vi "ProyectoEstacionamientoFINAL.vi"() -> ()   [LabVIEW 2020]
uses:
  <vilib>/Instr/_visa.llb/VISA Configure Serial Port (Instr).vi
panel:
  out "Lugar  6":string
  out "Lugar 5":string
  out "Lugar 4":string
  out "Lugar 3":string
  out "Lugar 2":string
  out "Lugar 1":string
  out "ESTACIONAMIENTO LLENO":bool
  out "Lugares ocupados":i32
  in  "SALIDA":bool
  in  "ENTRADA":bool
  in  "length (rest) 6":i32
  in  "offset (0) 6":i32
  out "Ocupación espacio 6":string
  out "cadena 6":dbl
  in  "length (rest) 5":i32
  in  "offset (0) 5":i32
  out "Ocupación espacio 5":string
  out "cadena 5":dbl
  in  "length (rest) 4":i32
  in  "offset (0) 4":i32
  out "Ocupación espacio 4":string
  out "cadena 4":dbl
  out "Ocupación espacio 3":string
  in  "length (rest) 3":i32
  in  "offset (0) 3":i32
  out "cadena 3":dbl
  in  "length (rest) 2":i32
  in  "offset (0) 2":i32
  out "Ocupación espacio 2":string
  out "cadena 2":dbl
  out "Ocupación espacio 1":string
  in  "length (rest)":i32
  in  "offset (0)":i32
  out "cadena 1":dbl
  in  "stop":bool
  in  "VISA resource name":refnum<visa-resource-name>
  # "Bienvenidos al estacionamiento de la UPIIZ"
  # "Toca el botón para continuar"
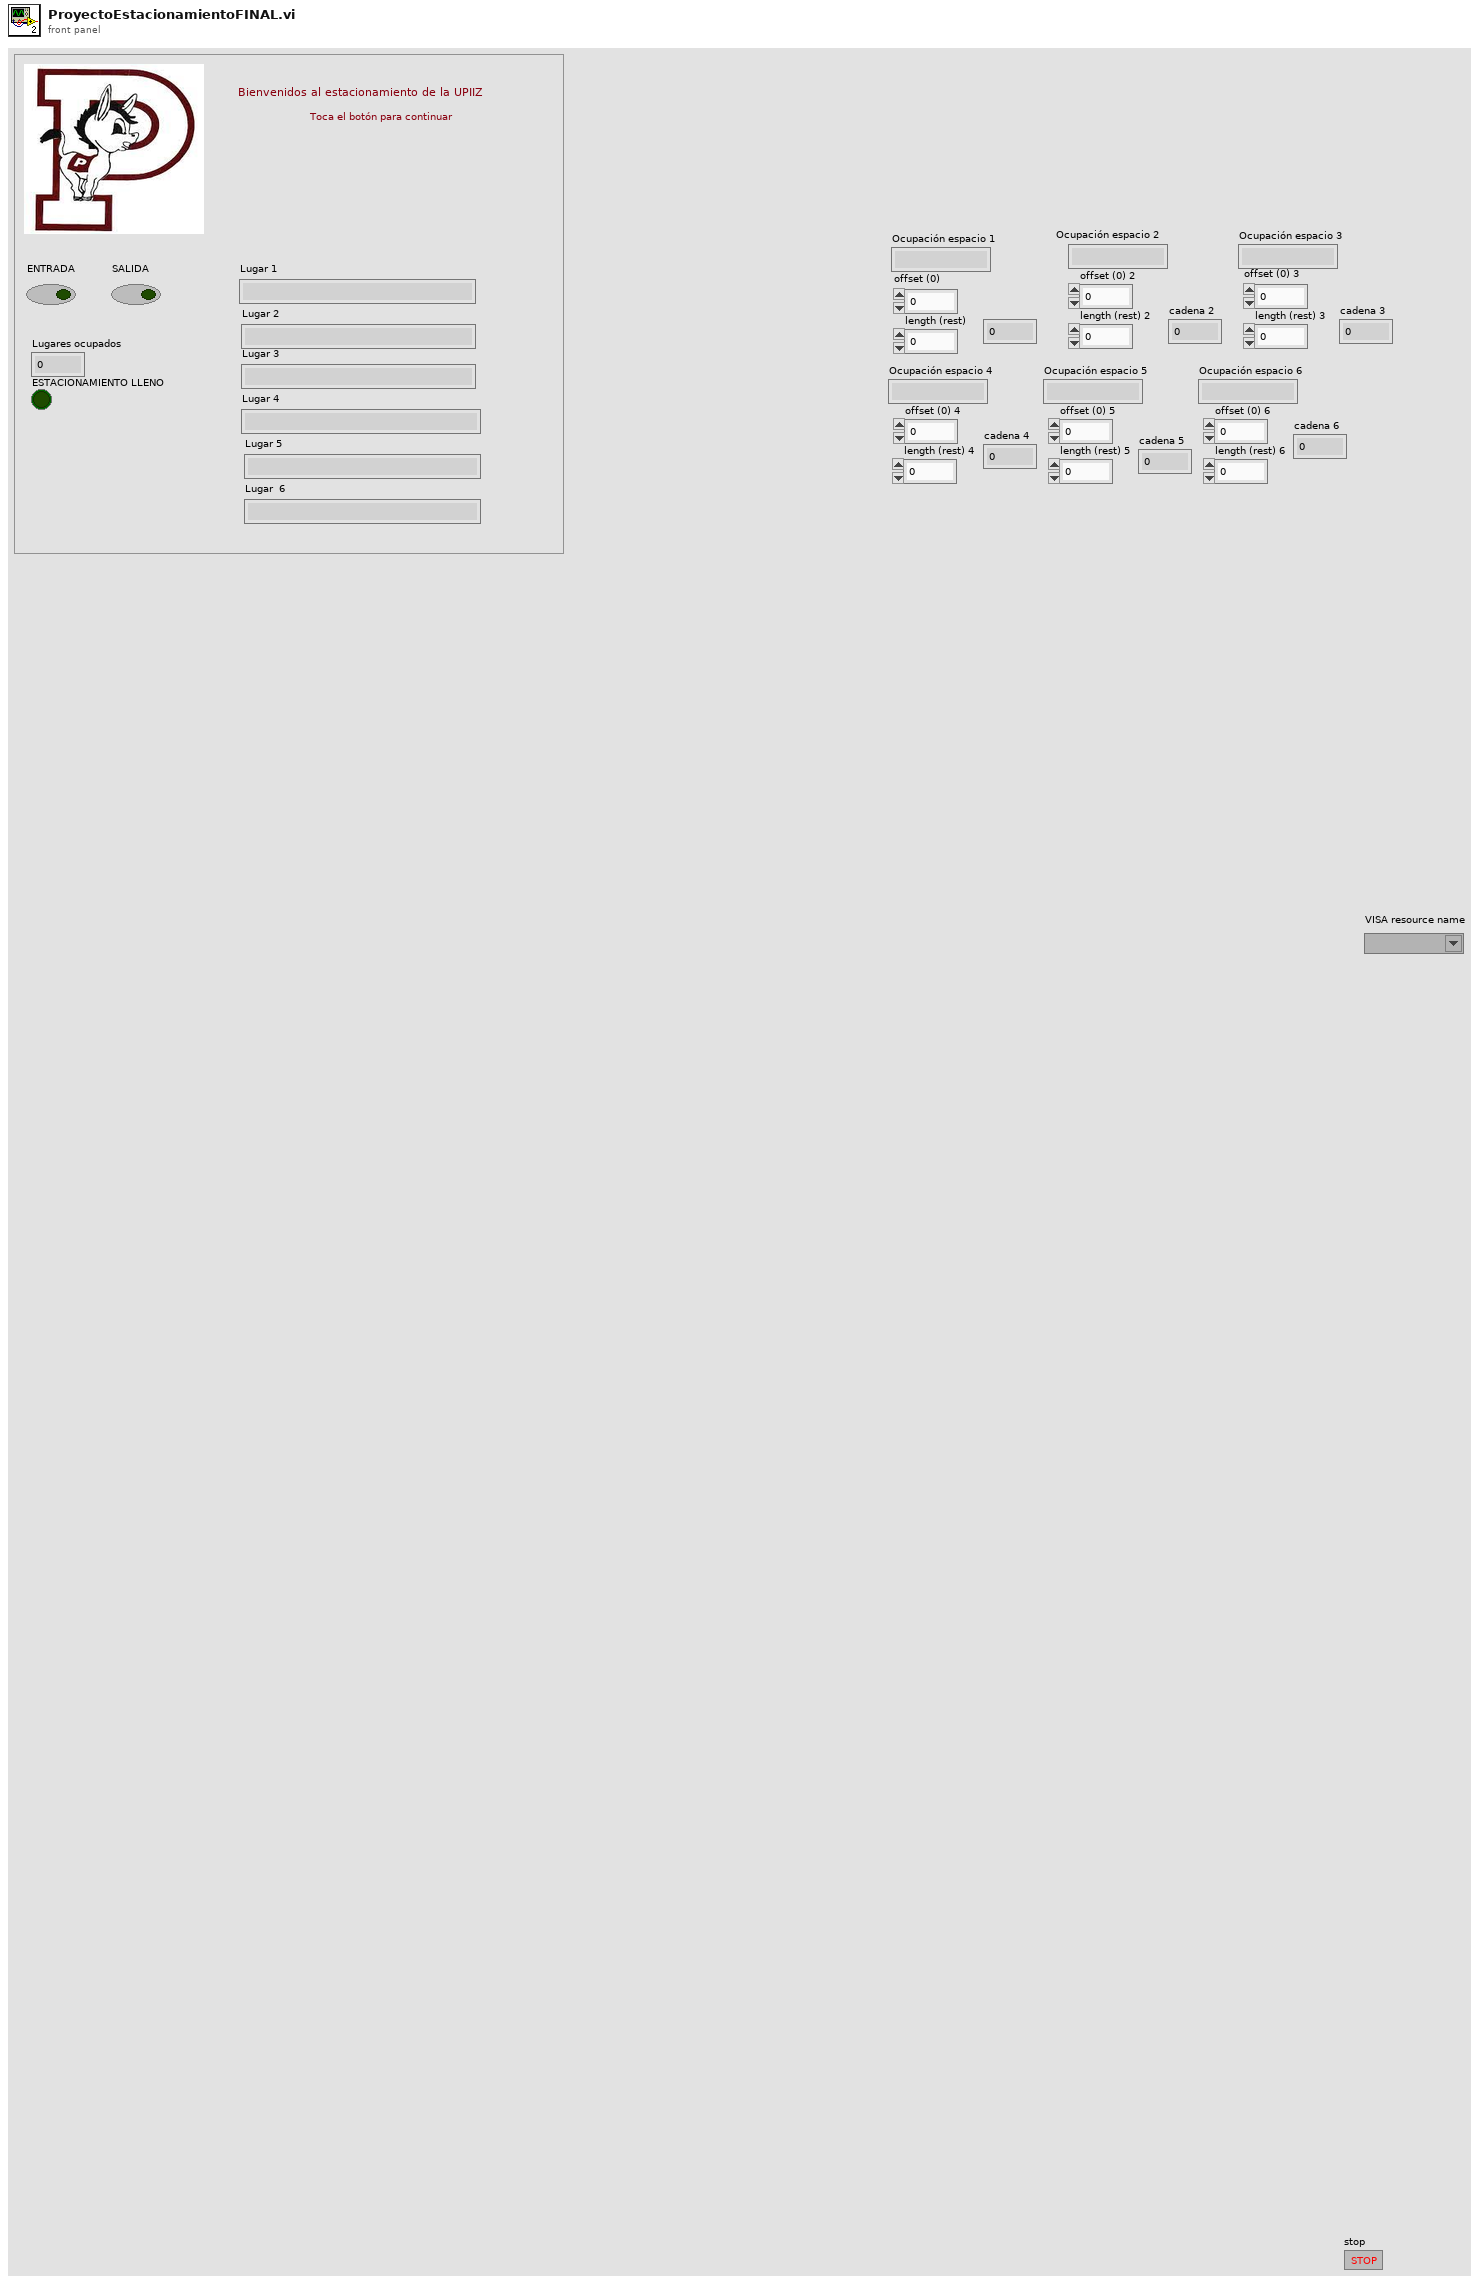
[diagram p1: front panel]
types:
  T1 = enum8{"Enabled", "Disabled", "Disabled and Grayed Out"}
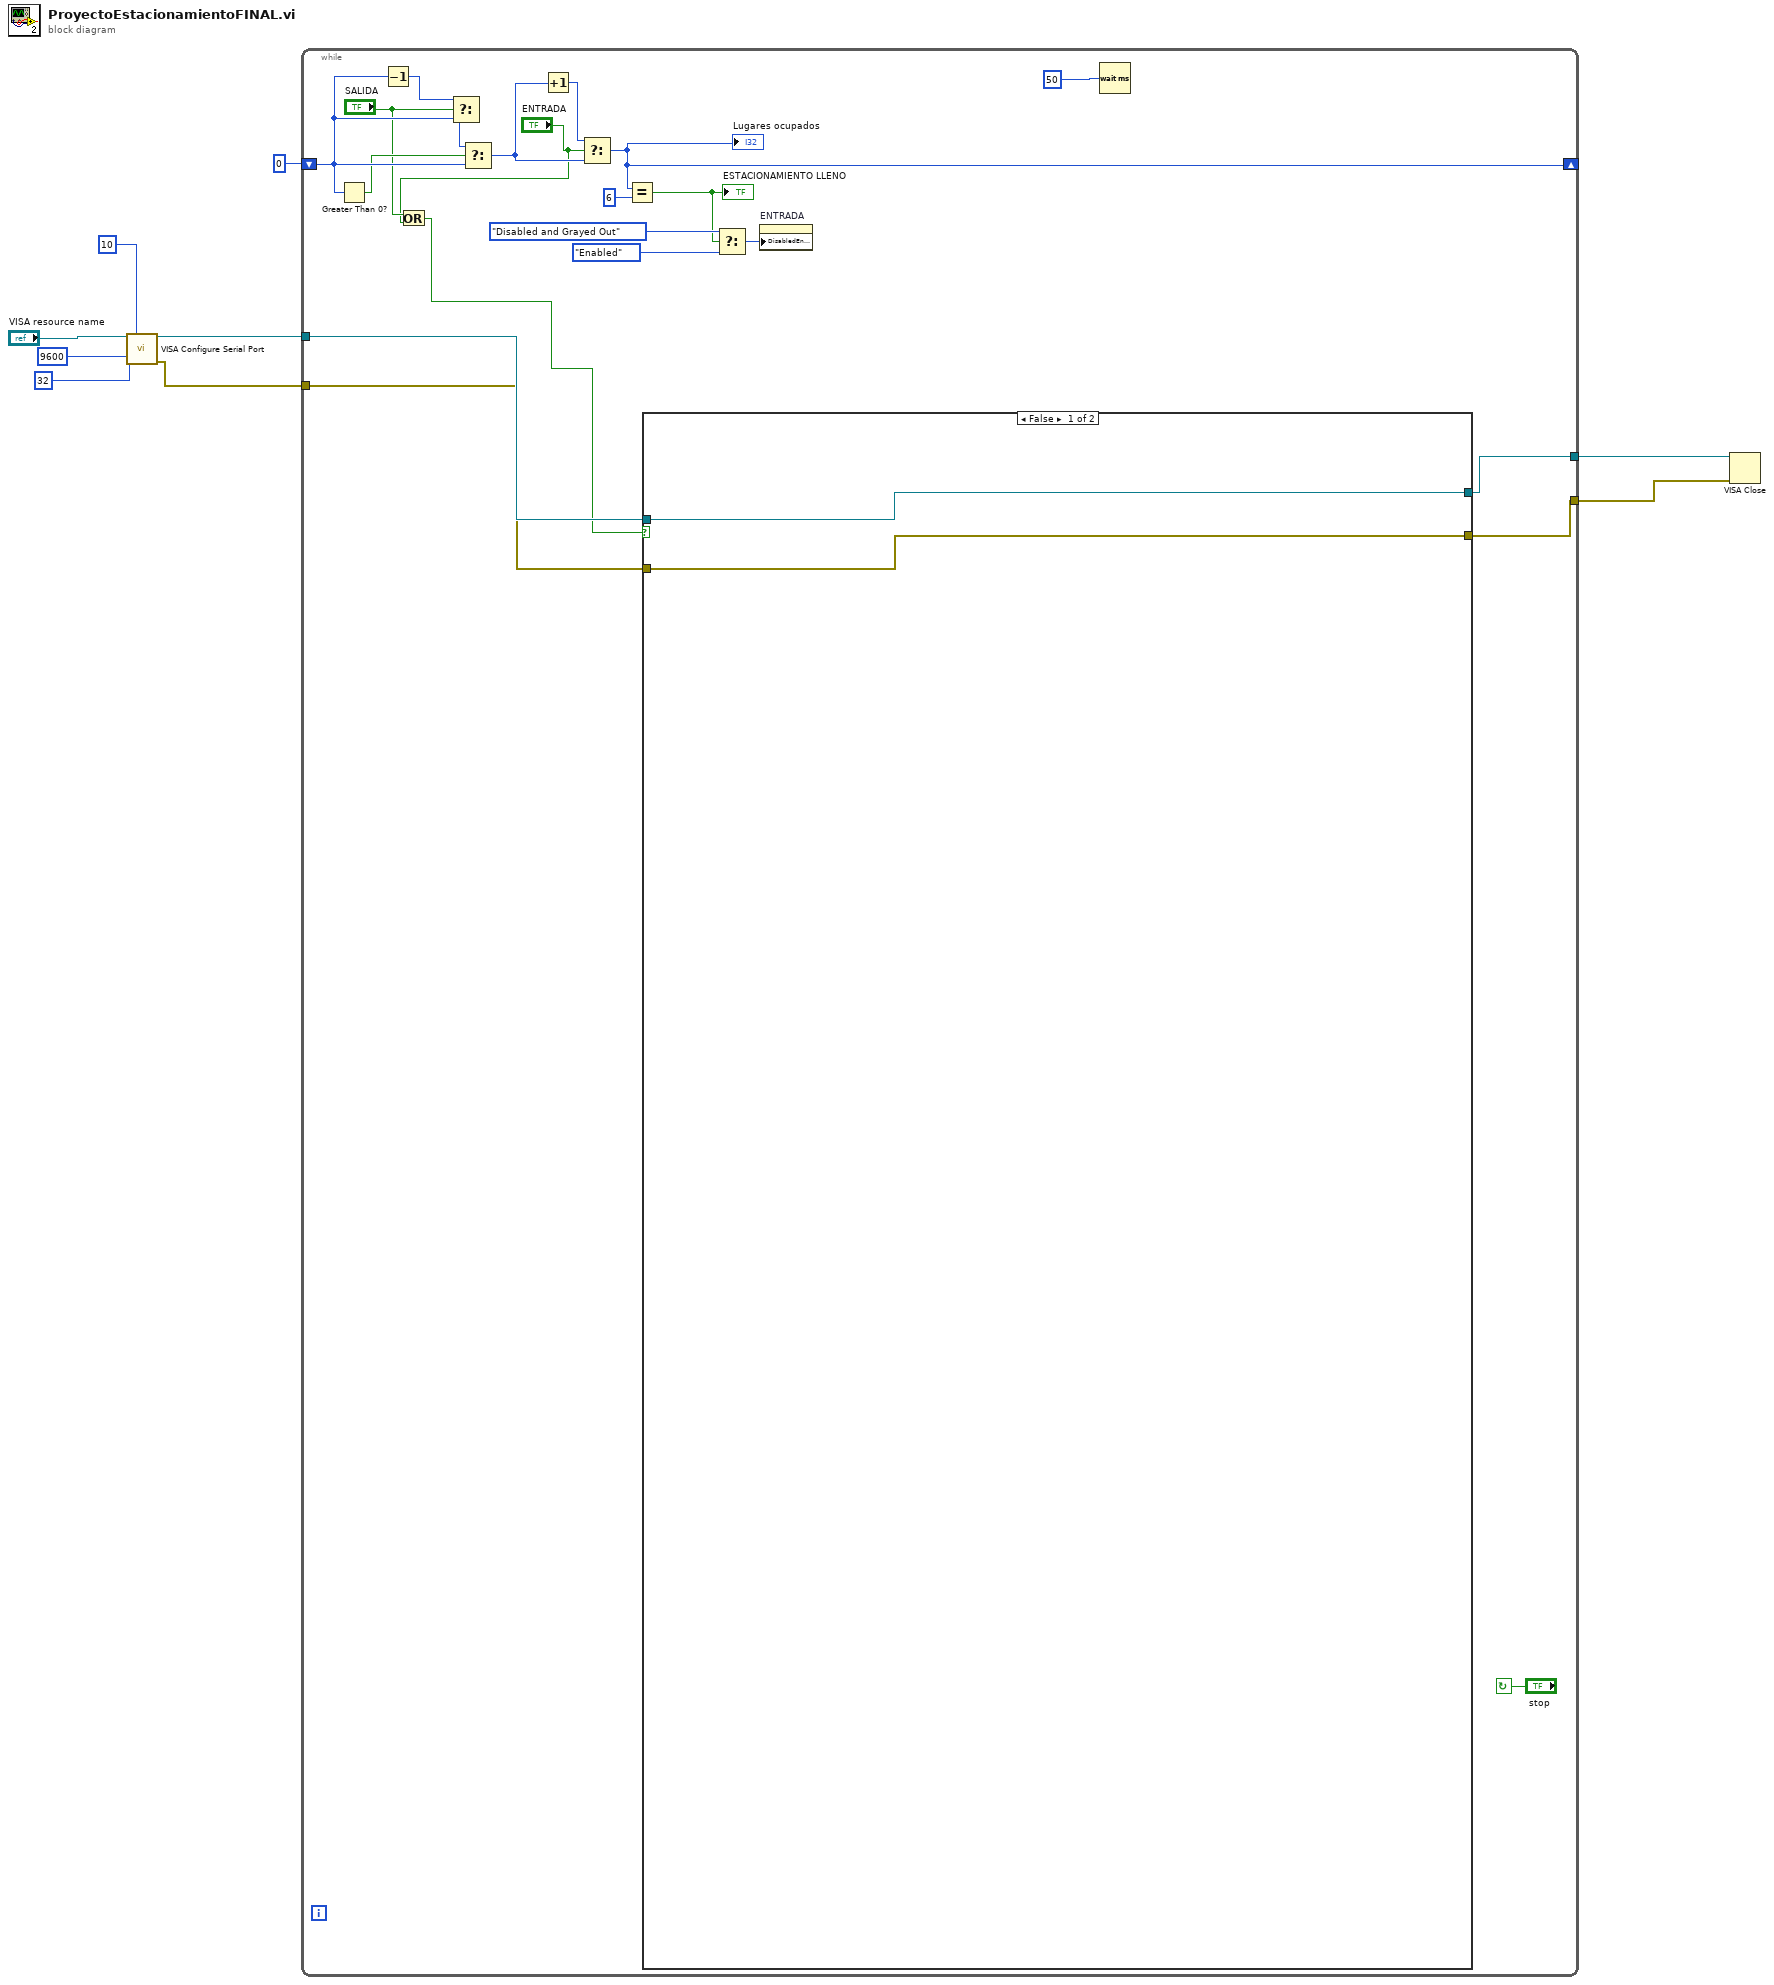
[diagram p0: block diagram]
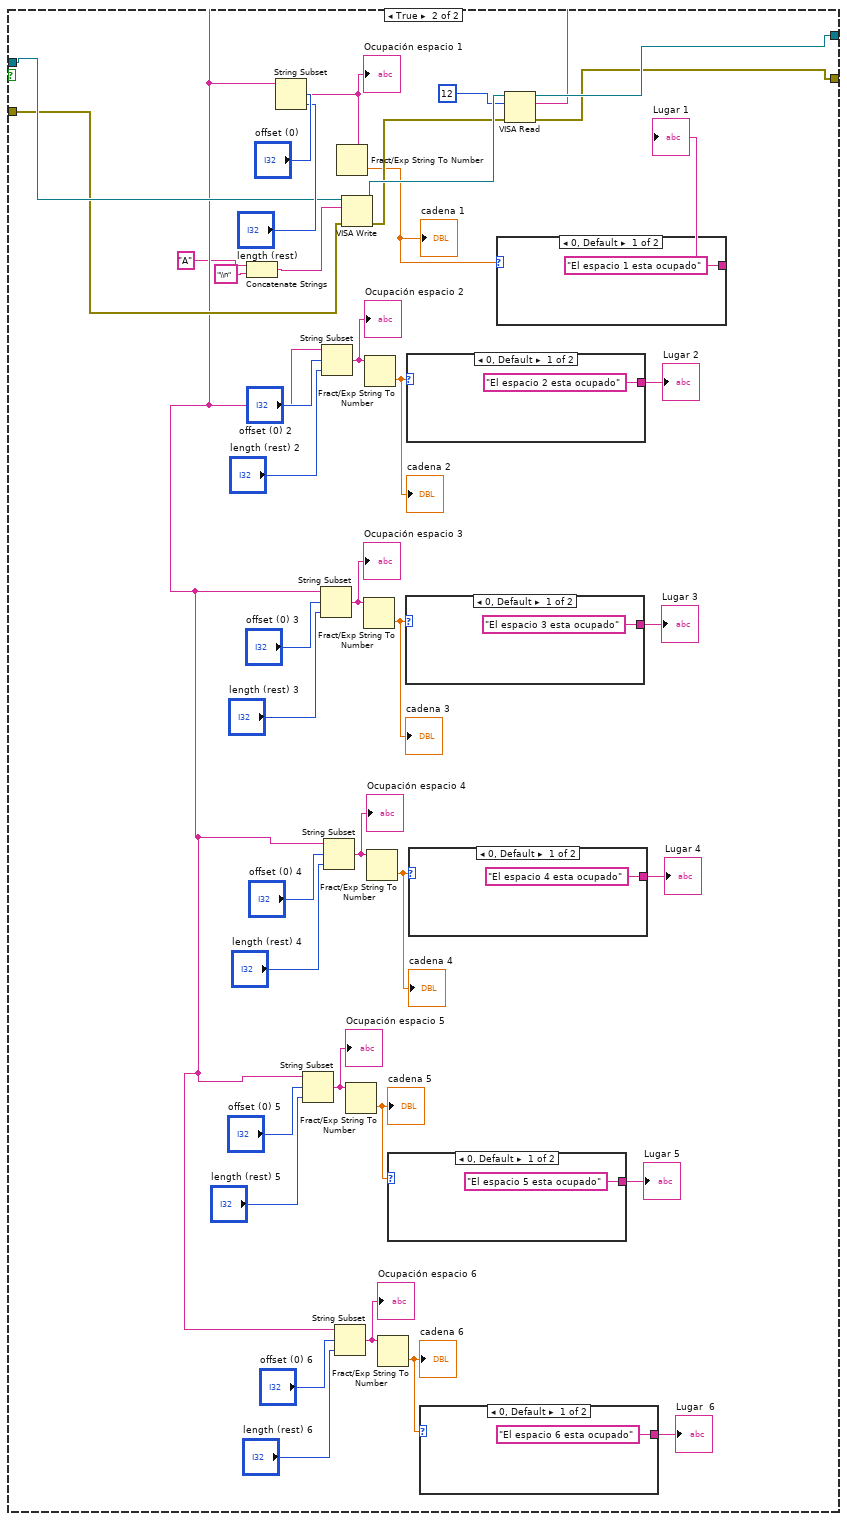
[diagram p2: hidden frame]
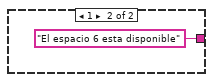
[diagram p3: hidden frame]
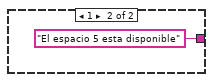
[diagram p4: hidden frame]
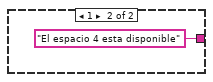
[diagram p5: hidden frame]
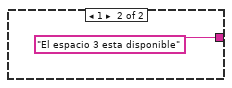
[diagram p6: hidden frame]
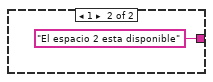
[diagram p7: hidden frame]
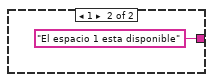
[diagram p8: hidden frame]
diagram:
  n1 = call-poly "VISA Configure Serial Port"("VISA resource name"="VISA resource name", "timeout (10sec)"=u32 10, "baud rate (9600)"=u32 9600, "data bits (8)"=u16 32) -> ("VISA resource name out"=w2:refnum<visa-resource-name>, "error out"=w4:errorcluster)  [unwired: 10 in]
  n2 = while {
    shift-right: [w27] -> _
    shift-left: 0 -> [w23]
    tunnel: w4 -> [w16]
    tunnel: [w13] -> w3
    tunnel: w2 -> [w17]
    tunnel: [w14] -> w1
    stop <- "stop" continue-if-true
    n3 = Greater Than 0?(x=w23) -> (x > 0?=w18:bool)
    n4 = Decrement(x=w23) -> (x-1=w28:i32)
    n5 = Or(x="SALIDA", y="ENTRADA") -> (x .or. y?=w10:bool)
    n6 = Select(t=w28, s="SALIDA", f=w23) -> (s? t:f=w25:i32)
    n7 = Select(t=w25, s=w18, f=w23) -> (s? t:f=w24:i32)
    n8 = Increment(x=w24) -> (x+1=w29:i32)
    n9 = Select(t=w29, s="ENTRADA", f=w24) -> (s? t:f=w27:i32)
    "Lugares ocupados" <- w27
    n10 = Equal?(x=w27, y=6) -> (x = y?=w19:bool)
    "ESTACIONAMIENTO LLENO" <- w19
    n11 = case shown="False" w10 {
      tunnel: w17 -> [w32 w38]
      tunnel: w16 -> [w31 w37]
      tunnel: [w31 w39] -> w13
      tunnel: [w32 w40] -> w14
      frame False {
      }
      frame True {
        n12 = Concatenate Strings("A" ("string"), "\\n" ("string")) -> (w35:string)
        n13 = VISA Write(VISA resource name=w38, write buffer=w35, error in (no error)=w37) -> (VISA resource name out=w73:refnum<visa-resource-name>, error out=w72:errorcluster)  [unwired: 1 out]
        n14 = VISA Read(VISA resource name=w73, byte count=u32 12, error in (no error)=w72) -> (VISA resource name out=w40:refnum<visa-resource-name>, read buffer=w36:string, error out=w39:errorcluster)  [unwired: 1 out]
        n15 = String Subset(string=w36, offset (0)="offset (0)", length (rest)="length (rest)") -> (substring=w66:string)
        "Ocupación espacio 1" <- w66
        n16 = String Subset(string=w36, offset (0)="offset (0) 5", length (rest)="length (rest) 5") -> (substring=w48:string)
        "Ocupación espacio 5" <- w48
        n17 = String Subset(string=w36, offset (0)="offset (0) 3", length (rest)="length (rest) 3") -> (substring=w56:string)
        "Ocupación espacio 3" <- w56
        n18 = String Subset(string=w36, offset (0)="offset (0) 2", length (rest)="length (rest) 2") -> (substring=w63:string)
        "Ocupación espacio 2" <- w63
        n19 = String Subset(string=w36, offset (0)="offset (0) 4", length (rest)="length (rest) 4") -> (substring=w53:string)
        "Ocupación espacio 4" <- w53
        n20 = String Subset(string=w36, offset (0)="offset (0) 6", length (rest)="length (rest) 6") -> (substring=w43:string)
        "Ocupación espacio 6" <- w43
        n21 = Fract/Exp String To Number(string=w66) -> (number=w68:dbl)  [unwired: 3 in, 1 out]
        "cadena 1" <- w68
        n22 = Fract/Exp String To Number(string=w48) -> (number=w47:dbl)  [unwired: 3 in, 1 out]
        "cadena 5" <- w47
        n23 = Fract/Exp String To Number(string=w56) -> (number=w58:dbl)  [unwired: 3 in, 1 out]
        "cadena 3" <- w58
        n24 = Fract/Exp String To Number(string=w63) -> (number=w62:dbl)  [unwired: 3 in, 1 out]
        "cadena 2" <- w62
        n25 = Fract/Exp String To Number(string=w53) -> (number=w52:dbl)  [unwired: 3 in, 1 out]
        "cadena 4" <- w52
        n26 = Fract/Exp String To Number(string=w43) -> (number=w42:dbl)  [unwired: 3 in, 1 out]
        "cadena 6" <- w42
        n27 = case shown="0, Default" w47 {
          tunnel: ["El espacio 5 esta ocupado" "El espacio 5 esta disponible"] -> w46
          frame 0, Default {
          }
          frame 1 {
          }
        }
        "Lugar 5" <- w46
        n28 = case shown="0, Default" w58 {
          tunnel: ["El espacio 3 esta ocupado" "El espacio 3 esta disponible"] -> w57
          frame 0, Default {
          }
          frame 1 {
          }
        }
        "Lugar 3" <- w57
        n29 = case shown="0, Default" w62 {
          tunnel: ["El espacio 2 esta ocupado" "El espacio 2 esta disponible"] -> w61
          frame 0, Default {
          }
          frame 1 {
          }
        }
        "Lugar 2" <- w61
        n30 = case shown="0, Default" w52 {
          tunnel: ["El espacio 4 esta ocupado" "El espacio 4 esta disponible"] -> w51
          frame 0, Default {
          }
          frame 1 {
          }
        }
        "Lugar 4" <- w51
        n31 = case shown="0, Default" w42 {
          tunnel: ["El espacio 6 esta ocupado" "El espacio 6 esta disponible"] -> w41
          frame 0, Default {
          }
          frame 1 {
          }
        }
        "Lugar  6" <- w41
        n32 = case shown="0, Default" w68 {
          tunnel: ["El espacio 1 esta ocupado" "El espacio 1 esta disponible"] -> w67
          frame 0, Default {
          }
          frame 1 {
          }
        }
        "Lugar 1" <- w67
      }
    }
    n33 = Select(t=T1."Disabled and Grayed Out" ("Disabled"), s=w19, f=T1."Enabled" ("Disabled")) -> (s? t:f=w22:T1)
    n34 = property on="ENTRADA" class="Bool"("DisabledEnum"=w22) -> ()  [unwired: 2 in, 2 out]
    n35 = Wait (ms)(milliseconds to wait=u32 50) -> ()  [unwired: 1 out]
  }
  n36 = VISA Close(VISA resource name=w1, error in (no error)=w3) -> ()  [unwired: 1 out]
